vi "Directory_Separator.vi"() -> (1 "Separator":string, 2 "Setup string":string)   [LabVIEW 2022 SP3]
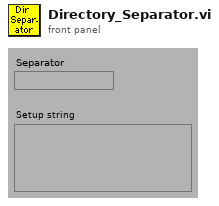
[diagram p1: front panel]
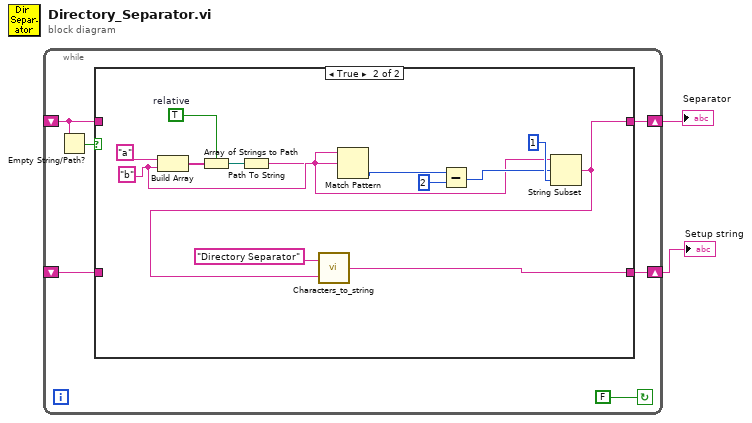
[diagram p0: block diagram]
diagram:
  n1 = while {
    shift-right: [w8] -> w2
    shift-left: _ -> [w5]
    shift-right: [w7] -> w1
    shift-left: _ -> [w4]
    stop <- FALSE continue-if-true
    n2 = Empty String/Path?(string/path=w5) -> (empty?=w6:bool)
    n3 = case shown="True" w6 {
      tunnel: [w10 w12] -> w8
      tunnel: [w9 w11] -> w7
      tunnel: w5 -> [w10 _]
      tunnel: w4 -> [w9 _]
      frame False {
      }
      frame True {
        w18 = TRUE  # relative
        w17 = "b"
        n4 = Build Array("a", w17) -> (w22:string[])
        n5 = Array of Strings to Path(0:w22, 1:w18) -> (2:w21:path)
        n6 = Path To String(path=w21) -> (string=w13:string)
        n7 = Match Pattern(string=w13, regular expression=w17) -> (offset past match=w16:i32)  [unwired: 4 out]
        n8 = Subtract(x=w16, y=2) -> (x-y=w14:i32)
        n9 = String Subset(string=w13, offset (0)=w14, length (rest)=1 ("length")) -> (substring=w12:string)
        n10 = call "Characters_to_string.vi"("Characters to write"=w12, "Label for characters"="Directory Separator") -> ("Output string"=w11:string)  [unwired: 1 in]
      }
    }
  }
  "Separator" <- w2
  "Setup string" <- w1
